vi "LV_Analog_IN.vi"() -> ()   [LabVIEW 2014]
uses:
  <vilib>/Instr/_visa.llb/VISA Configure Serial Port (Instr).vi
  <vilib>/ptbypt/NI_PtbyPt.lvlib
panel:
  out "Waveform Chart":dbl[](graph)
  in  "VISA resource name":refnum<visa-resource-name>
  in  "Stop Button":bool
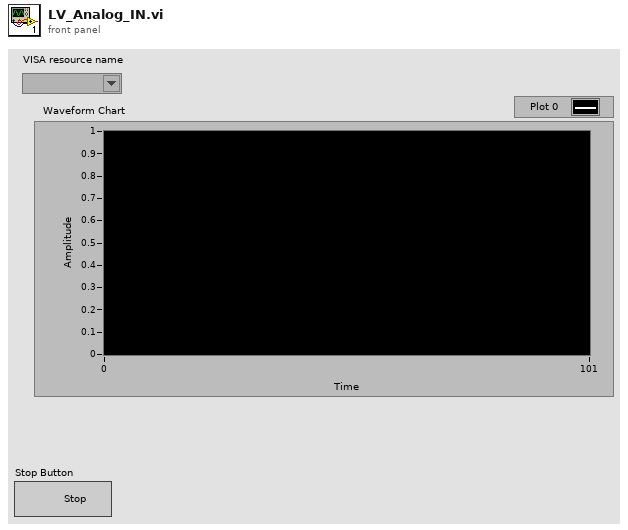
[diagram p1: front panel]
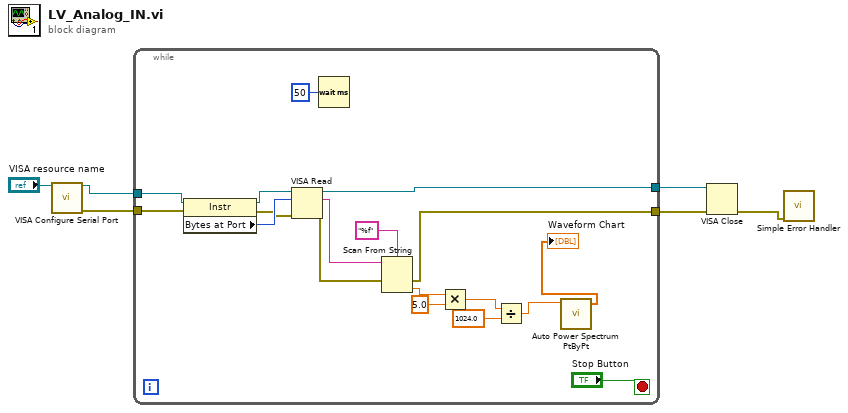
[diagram p0: block diagram]
diagram:
  n1 = call-poly "VISA Configure Serial Port"("VISA resource name"="VISA resource name") -> ("VISA resource name out"=w6:refnum<visa-resource-name>, "error out"=w3:errorcluster)  [unwired: 13 in]
  n2 = while {
    tunnel: w6 -> [w22]
    tunnel: [w23] -> w5
    tunnel: w3 -> [w13]
    tunnel: [w10] -> w2
    stop <- "Stop Button" stop-if-true
    n3 = property class="Instr"(reference=w22, error in=w13) -> (reference out=w21:refnum<visa-resource-name>, error out=w12:errorcluster, "Bytes at Port"=w20:u32)
    n4 = VISA Read(VISA resource name=w21, byte count=w20, error in (no error)=w12) -> (VISA resource name out=w23:refnum<visa-resource-name>, read buffer=w19:string, error out=w11:errorcluster)  [unwired: 1 out]
    n5 = Wait (ms)(milliseconds to wait=u32 50) -> ()  [unwired: 1 out]
    n6 = Scan From String(format string="%f", input string=w19, error in=w11) -> (error out=w10:errorcluster, output 1=w17:dbl)  [unwired: 2 in, 2 out]
    n7 = Multiply(x=w17, y=5.0) -> (x*y=w15:dbl)
    n8 = Divide(x=w15, y=1024.0) -> (x/y=w8:dbl)
    n9 = call <vilib>:"Auto Power Spectrum PtByPt.vi"("signal"=w8) -> ("Power Spectrum (V^2 rms)"=→"Waveform Chart":dbl[])  [unwired: 4 in, 2 out]
  }
  n10 = VISA Close(VISA resource name=w5, error in (no error)=w2) -> (error out=w1:errorcluster)
  n11 = call <vilib>:"Simple Error Handler.vi"("error in (no error)"=w1) -> ()  [unwired: 4 in, 5 out]
